vi "Set Voltage.vi"(8 "error in":errorcluster, 10 "V":dbl, 11 "DAQ HVPS in":refnum<class "DAQ HVPS.lvclass">) -> (0 "error out":errorcluster, 3 "DAQ HVPS out":refnum<class "DAQ HVPS.lvclass">)   [LabVIEW 2014, in "DAQ HVPS.lvclass"]
uses:
  DAQ HVPS.lvclass
  DAQ HVPS.lvclass/DAQ HVPS.ctl
  Base/Session HVPS.lvclass/Session HVPS.ctl
  Base/Write Vsp.vi
  <vilib>/DAQmx/write.llb/DAQmx Write (Analog DBL 1Chan 1Samp).vi
  <resource>/objmgr/daqmx.rc
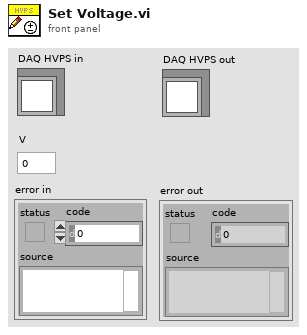
[diagram p1: front panel]
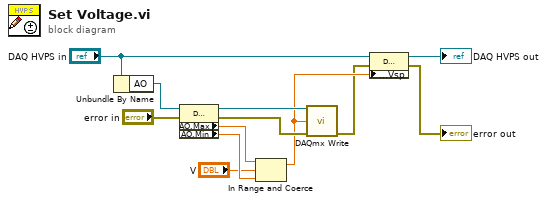
[diagram p0: block diagram]
diagram:
  n1 = Unbundle By Name("DAQ HVPS in") -> ("AO"=w9:refnum<k21>)
  n2 = property class="DAQmx Channel"(reference=w9, error in="error in") -> (reference out=w4:refnum<k21>, error out=w5:errorcluster, "AO.Max"=w8:dbl, "AO.Min"=w7:dbl)
  n3 = In Range and Coerce(upper limit=w8, x="V", lower limit=w7) -> (coerced(x)=w3:dbl)  [unwired: 1 out]
  n4 = call-poly <vilib>:"DAQmx Write.vi"("task/channels in"=w4, "data"=w3, "error in"=w5) -> ("error out"=w2:errorcluster)  [unwired: 10 in, 2 out]
  n5 = property class="DAQ HVPS"(reference="DAQ HVPS in", error in=w2, "Accessors:Vsp"=w3) -> (reference out=→"DAQ HVPS out":refnum<class "DAQ HVPS.lvclass">, error out=→"error out":errorcluster)
